vi "Perform_large_file_Analysis - Copy.vi"(7 "error in":errorcluster) -> (2 "Wvfm":waveform(dbl)[](array[waveform]), 5 "Nb of Events":dbl)   [LabVIEW 2019]
uses:
  <vilib>/Utility/error.llb/DialogType.ctl
  ESA_Data_Analysis_Global_VIs.vi
  SiPM_Tests_Global_Var.vi
panel:
  out "size(s) 2":i32
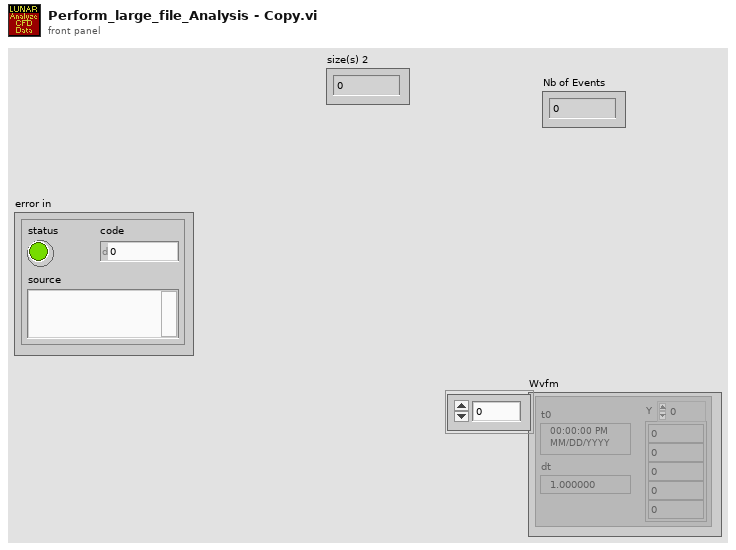
[diagram p1: front panel]
types:
  T1 = typedef "DialogType.ctl" = u16
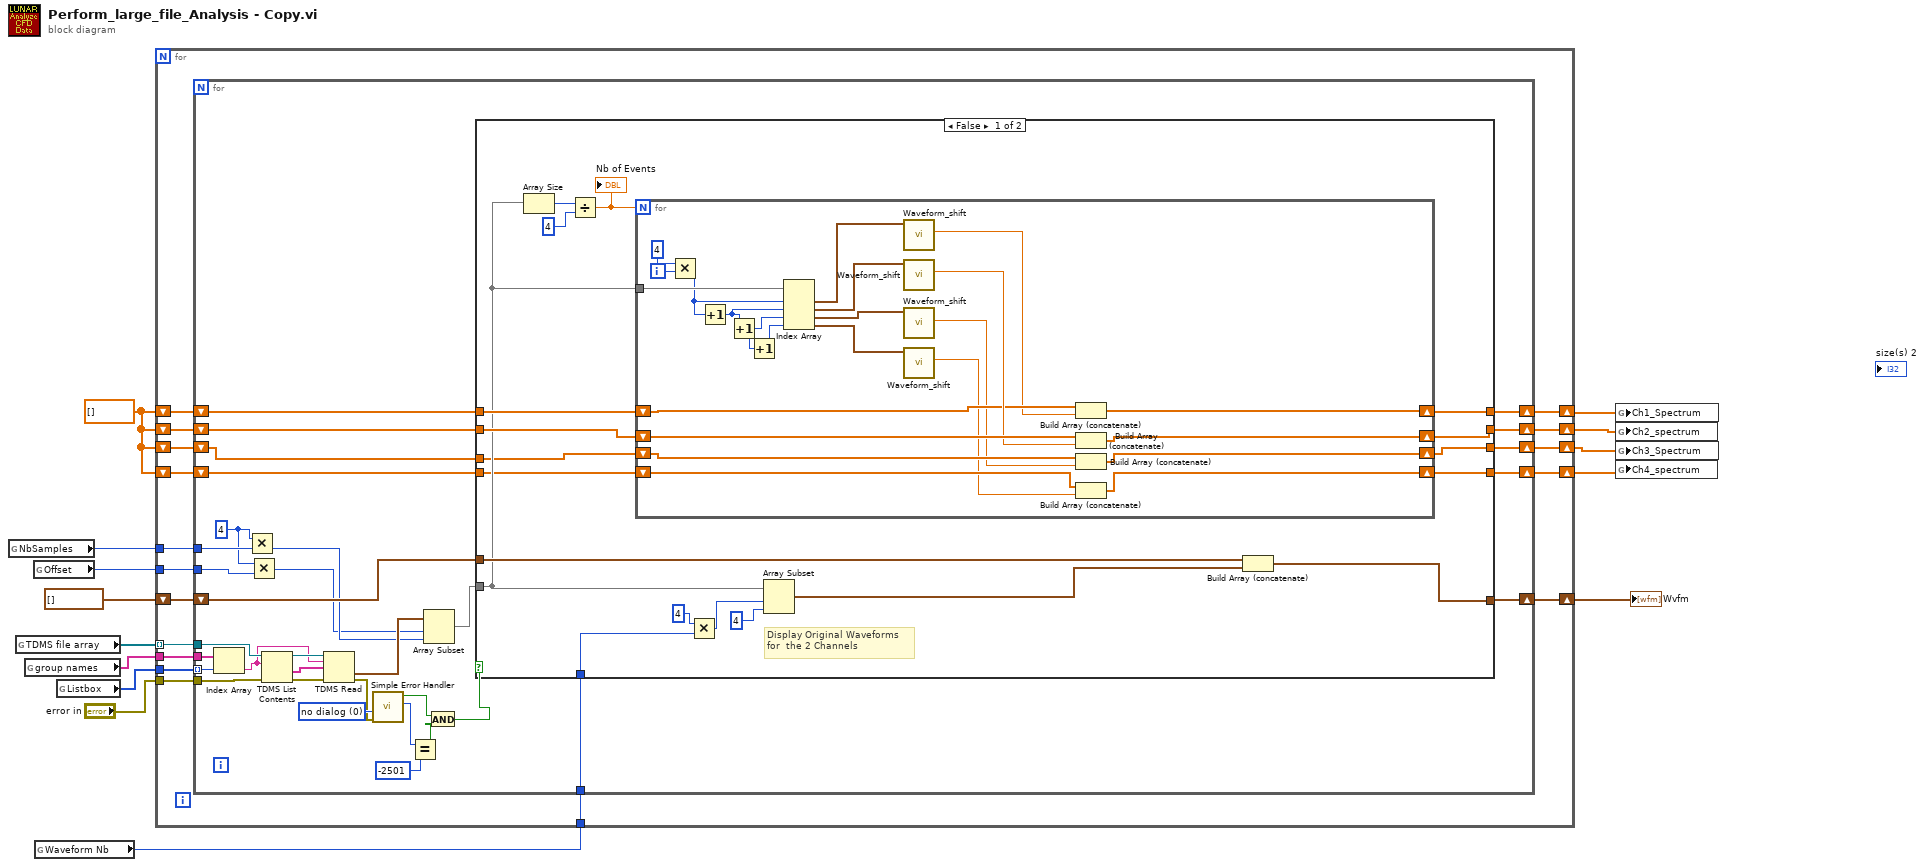
[diagram p0: block diagram]
diagram:
  w3 = dbl[] []
  n1 = global read "SiPM_Tests_Global_Var.vi" "NbSamples"() -> (w7:i64)
  n2 = global read "SiPM_Tests_Global_Var.vi" "TDMS file array"() -> (w11:refnum<k34>[])
  n3 = global read "ESA_Data_Analysis_Global_VIs.vi" "group names"() -> (w14:string[])
  n4 = global read "SiPM_Tests_Global_Var.vi" "Offset"() -> (w9:i64)
  n5 = global read "SiPM_Tests_Global_Var.vi" "Waveform Nb"() -> (w6:u16)
  n6 = global read "ESA_Data_Analysis_Global_VIs.vi" "Listbox"() -> (w13:i32[])
  n7 = for {
    tunnel: w11 -> [w31] mode=indexing
    tunnel: w14 -> [w30]
    tunnel: w13 -> [w29]
    tunnel: "error in" -> [w28]
    tunnel: w9 -> [w26]
    shift-right: [w27] -> w10
    shift-left: waveform(dbl)[] [] -> [w25]
    shift-right: [w21] -> w4
    shift-left: w3 -> [w24]
    shift-right: [w22] -> w5
    shift-left: w3 -> [w23]
    tunnel: w7 -> [w20]
    tunnel: w6 -> [w19]
    shift-right: [w16] -> w2
    shift-left: w3 -> [w18]
    shift-right: [w15] -> w1
    shift-left: w3 -> [w17]
    n8 = for {
      tunnel: w31 -> [w64]
      tunnel: w30 -> [w63]
      tunnel: w29 -> [w62] mode=indexing
      tunnel: w28 -> [w61]
      tunnel: w26 -> [w41]
      shift-right: [w54] -> w27
      shift-left: w25 -> [w53]
      shift-right: [w44] -> w21
      shift-left: w24 -> [w47]
      shift-right: [w45] -> w22
      shift-left: w23 -> [w46]
      tunnel: w20 -> [w40]
      tunnel: w19 -> [w43]
      shift-right: [w33] -> w16
      shift-left: w18 -> [w35]
      shift-right: [w32] -> w15
      shift-left: w17 -> [w34]
      w36 = i64 4 ("x")
      w58 = T1 0 items=["no dialog", "OK message", "continue or stop message", "OK message + warnings", "continue/stop + warnings"] ("type of dialog (OK msg:1)")
      n9 = Index Array(array=w63, index=w62) -> (element=w59:string)
      n10 = Multiply(x=w36, y=w40) -> (x*y=w38:i64)
      n11 = Multiply(x=w36, y=w41) -> (x*y=w37:i64)
      n12 = TDMS List Contents(4:w61, 6:w59, 7:w64) -> (0:w55:errorcluster, 1:w56:string[], 3:w60:refnum<k34>)  [unwired: 1 out]
      n13 = TDMS Read(0:w60, 5:w59, 7:w56, 11:w55) -> (10:w42:waveform(dbl)[], 15:w57:errorcluster)  [unwired: 4 in, 4 out]
      n14 = call <vilib>:"Simple Error Handler.vi"("type of dialog (OK msg:1)"=w58, "error in (no error)"=w57) -> ("error?"=w51:bool, "code out"=w50:i32)  [unwired: 3 in, 3 out]
      n15 = Equal?(x=w50, y=-2501) -> (x = y?=w48:bool)
      n16 = Array Subset(array=w42, index=w37, length=w38) -> (w39:waveform(dbl)[])
      n17 = And(x=w51, y=w48) -> (x .and. y?=w52:bool)
      n18 = case shown="False" w52 {
        tunnel: w39 -> [w69 _]
        tunnel: [w82 w111] -> w54
        tunnel: w53 -> [w81 w111]
        tunnel: w47 -> [w77 w109]
        tunnel: w46 -> [w76 w110]
        tunnel: [w75 w110] -> w45
        tunnel: [w74 w109] -> w44
        tunnel: w43 -> [w70 _]
        tunnel: w35 -> [w68 w108]
        tunnel: w34 -> [w67 w107]
        tunnel: [w66 w108] -> w33
        tunnel: [w65 w107] -> w32
        frame False {
          # "Display Original Waveforms\nfor  the 2 Channels"
          n19 = Array Size(array=w69) -> (size(s)=w80:i32)
          n20 = Divide(x=w80, y=4) -> (x/y=w78:dbl)
          "Nb of Events" <- w78
          n21 = for {
            N: w78 -> [_]
            tunnel: w69 -> [w106]
            shift-right: [w92] -> w75
            shift-left: w76 -> [w93]
            shift-right: [w90] -> w74
            shift-left: w77 -> [w101]
            shift-right: [w87] -> w66
            shift-left: w68 -> [w89]
            shift-right: [w86] -> w65
            shift-left: w67 -> [w85]
            i -> [w100]
            n22 = Multiply(x=4, y=w100) -> (x*y=w104:i32)
            n23 = Increment(x=w104) -> (x+1=w98:i32)
            n24 = Increment(x=w98) -> (x+1=w96:i32)
            n25 = Increment(x=w96) -> (x+1=w97:i32)
            n26 = Index Array(array=w106, index #1=w104, index #2=w98, index #3=w96, index #4=w97) -> (element #1=w103:waveform(dbl), element #2=w102:waveform(dbl), element #3=w95:waveform(dbl), element #4=w94:waveform(dbl))
            n27 = call "Waveform_shift.vi"("Waveform_in"=w103) -> ("Peak Value"=w91:dbl)  [unwired: 9 in]
            n28 = call "Waveform_shift.vi"("Waveform_in"=w102) -> ("Peak Value"=w99:dbl)  [unwired: 9 in]
            n29 = call "Waveform_shift.vi"("Waveform_in"=w95) -> ("Peak Value"=w88:dbl)  [unwired: 9 in]
            n30 = call "Waveform_shift.vi"("Waveform_in"=w94) -> ("Peak Value"=w84:dbl)  [unwired: 9 in]
            n31 = Build Array (concatenate)(w93, w91) -> (w92:dbl[])
            n32 = Build Array (concatenate)(w101, w99) -> (w90:dbl[])
            n33 = Build Array (concatenate)(w89, w88) -> (w87:dbl[])
            n34 = Build Array (concatenate)(w85, w84) -> (w86:dbl[])
          }
          n35 = Multiply(x=4, y=w70) -> (x*y=w73:i32)
          n36 = Array Subset(array=w69, index=w73, length=4) -> (w83:waveform(dbl)[])
          n37 = Build Array (concatenate)(w81, w83) -> (w82:waveform(dbl)[])
        }
        frame True {
        }
      }
    }
  }
  "Wvfm" <- w10
  n38 = global write "SiPM_Tests_Global_Var.vi" "Ch1_Spectrum"(w5) -> ()
  n39 = global write "SiPM_Tests_Global_Var.vi" "Ch2_spectrum"(w4) -> ()
  n40 = global write "SiPM_Tests_Global_Var.vi" "Ch3_Spectrum"(w2) -> ()
  n41 = global write "SiPM_Tests_Global_Var.vi" "Ch4_spectrum"(w1) -> ()
